vi "Check Status.vi"(8 "error in (no error)":errorcluster, 11 "Lockin and Fluke Multimeter in":refnum<class "Lockin and Fluke Multimeter.lvclass">) -> (0 "error out":errorcluster, 1 "Status":string, 2 "Ready?":bool, 3 "Lockin and Fluke Multimeter out":refnum<class "Lockin and Fluke Multimeter.lvclass">)   [LabVIEW 2023, in "Lockin and Fluke Multimeter.lvclass"]
doc: "(Dynamic) Check if the instrument is powered on and update its member fields with the instrument's current status. Optionally return a text status message."
uses:
  Lockin and Fluke Multimeter.lvclass
  Lockin and Fluke Multimeter.lvclass/Lockin and Fluke Multimeter.ctl
  Utility Classes/Readable/Readable.lvclass
  Lockin/sr830/SR830.lvlib
  Fluke Multimeter/Fluke 8840/Fluke 8840.lvlib
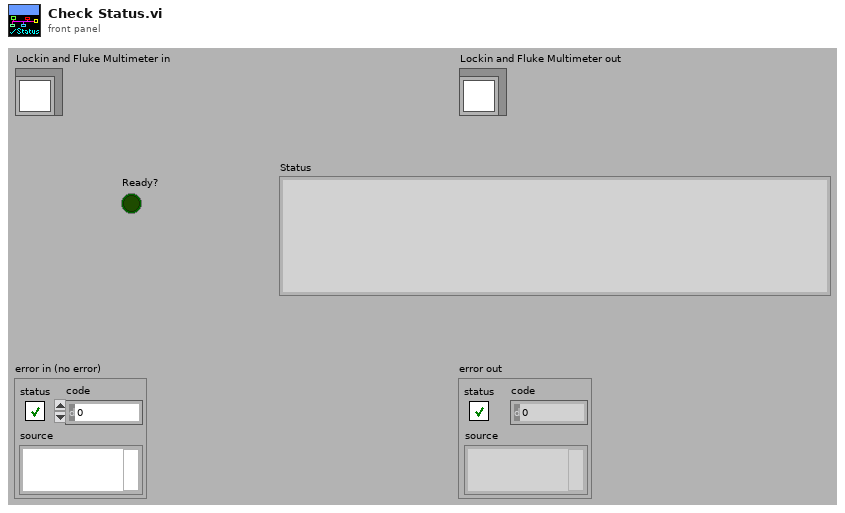
[diagram p1: front panel]
types:
  T1 = typedef "SR830.lvlib/Sensitivity_in_library.ctl" = u16
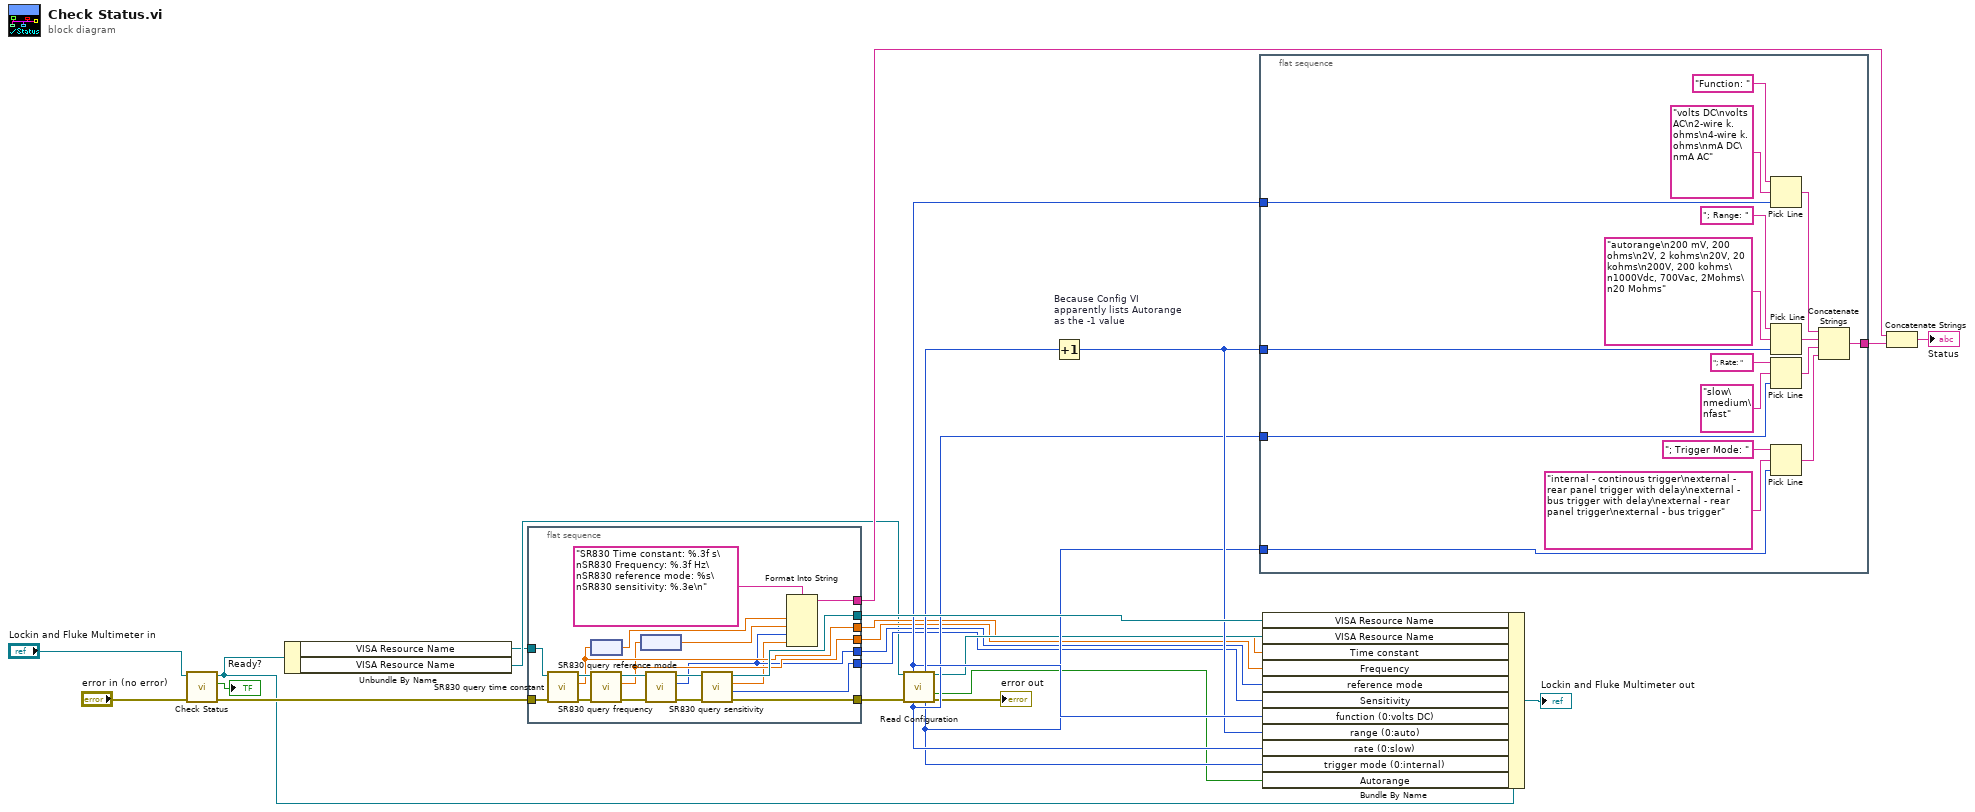
[diagram p0: block diagram]
diagram:
  n1 = call-parent "Check Status.vi"("error in (no error)"="error in (no error)", "Instrument in"="Lockin and Fluke Multimeter in") -> ("error out"=w22:errorcluster, "Ready?"=→"Ready?":bool, "Instrument out"=w21:refnum<class "Lockin and Fluke Multimeter.lvclass">)  [unwired: 6 in, 1 out]
  n2 = Unbundle By Name(w21) -> ("VISA Resource Name"=w1:refnum<visa-resource-name>, "VISA Resource Name"=w2:refnum<visa-resource-name>)
  n3 = flat-sequence {
    tunnel: w1 -> [w38]
    tunnel: w22 -> [w37]
    tunnel: [w36] -> w19
    tunnel: [w32] -> w17
    tunnel: [w31] -> w10
    tunnel: [w30] -> w6
    tunnel: [w29] -> w5
    tunnel: [w28] -> w4
    tunnel: [w27] -> w3
    frame #0 {
      n4 = call "SR830 query time constant.vi"("error in (no error)"=w37, "VISA resource name"=w38) -> ("error out"=w41:errorcluster, "time constant"=w30:dbl[unit], "VISA resource name out"=w39:refnum<visa-resource-name>)  [unwired: 7 in]
      n5 = node(w30) -> (w34:dbl)
      n6 = call "SR830 query frequency.vi"("error in (no error)"=w41, "VISA resource name"=w39) -> ("error out"=w42:errorcluster, "frequency"=w29:dbl[unit], "VISA resource name out"=w40:refnum<visa-resource-name>)  [unwired: 7 in]
      n7 = node(w29) -> (w33:dbl)
      n8 = call "SR830 query reference mode.vi"("error in (no error)"=w42, "VISA resource name"=w40) -> ("error out"=w44:errorcluster, "reference mode"=w28:enum16{"external", "internal"}, "VISA resource name out"=w43:refnum<visa-resource-name>)  [unwired: 7 in]
      n9 = call "SR830 query sensitivity.vi"("error in (no error)"=w44, "VISA resource name"=w43) -> ("error out"=w32:errorcluster, "Sensitivity"=w27:T1, "sensitivity"=w26:dbl[unit], "VISA resource name out"=w36:refnum<visa-resource-name>)  [unwired: 6 in]
      n10 = Format Into String(format string="SR830 Time constant: %.3f s\nSR830 Frequency: %.3f Hz\nSR830 reference mode: %s\nSR830 sensitivity: %.3e\n", w34, w33, w28, w26) -> (resulting string=w31:string)  [unwired: 2 in, 1 out]
    }
  }
  n11 = call "Read Configuration.vi"("VISA resource name"=w2, "error in (no error)"=w17) -> ("function"=w16:i32, "range"=w18:i32, "VISA resource name out"=w7:refnum<visa-resource-name>, "autorange"=w12:bool, "rate"=w14:i32, "trigger mode"=w13:i32, "error out"=→"error out":errorcluster)  [unwired: 7 out]
  n12 = Increment "Because Config VI\napparently lists Autorange\nas the -1 value"(x=w18) -> (x+1=w15:i32)
  n13 = flat-sequence {
    tunnel: [w59] -> w11
    tunnel: w16 -> [w57]
    tunnel: w15 -> [w54]
    tunnel: w14 -> [w49]
    tunnel: w13 -> [w48]
    frame #0 {
      n14 = Pick Line(string ("")="Function: ", multi-line string="volts DC\nvolts AC\n2-wire k.ohms\n4-wire k.ohms\nmA DC\nmA AC", line index=w57) -> (output string=w60:string)
      n15 = Pick Line(string ("")="; Range: ", multi-line string="autorange\n200 mV, 200 ohms\n2V, 2 kohms\n20V, 20 kohms\n200V, 200 kohms\n1000Vdc, 700Vac, 2Mohms\n20 Mohms", line index=w54) -> (output string=w53:string)
      n16 = Pick Line(string ("")="; Rate: ", multi-line string="slow\nmedium\nfast", line index=w49) -> (output string=w46:string)
      n17 = Pick Line(string ("")="; Trigger Mode: ", multi-line string="internal - continous trigger\nexternal - rear panel trigger with delay\nexternal - bus trigger with delay\nexternal - rear panel trigger\nexternal - bus trigger", line index=w48) -> (output string=w45:string)
      n18 = Concatenate Strings(w60, w53, w46, w45) -> (w59:string)
    }
  }
  n19 = Bundle By Name(cluster=w21, "VISA Resource Name"=w19, "VISA Resource Name"=w7, "Time constant"=w6, "Frequency"=w5, "reference mode"=w4, "Sensitivity"=w3, "function (0:volts DC)"=w16, "range (0:auto)"=w15, "rate (0:slow)"=w14, "trigger mode (0:internal)"=w13, "Autorange"=w12) -> (→"Lockin and Fluke Multimeter out":refnum<class "Lockin and Fluke Multimeter.lvclass">)
  n20 = Concatenate Strings(w10, w11) -> (→"Status":string)
